vi "Sets the ACW voltage for MANU.vi"(5 "Enable to Query":bool, 7 "Enable to Setup":bool, 8 "error in":errorcluster, 10 "ACW voltage(kV)":sgl=0.1 min=0.1 max=5 format="%.3f", 11 "VISA resource name":refnum<visa-resource-name>) -> (0 "error out":errorcluster, 2 "Return ACW voltage":string, 3 "VISA resource name out":refnum<visa-resource-name>)   [LabVIEW 2011, in "GPT-9000.lvlib"]
uses:
  <instrlib>/GPT-9000/GPT-9000.lvlib
panel:
  # "kV"
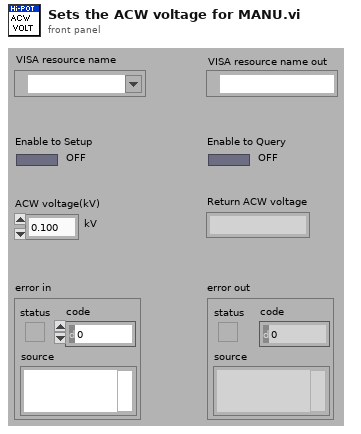
[diagram p1: front panel]
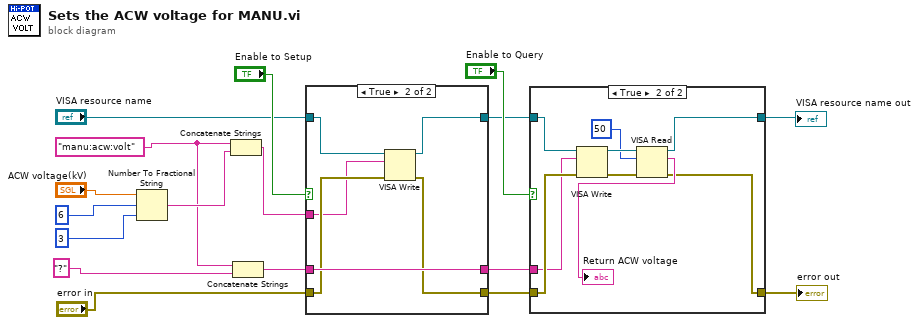
[diagram p0: block diagram]
diagram:
  w12 = "manu:acw:volt"
  n1 = Number To Fractional String(number="ACW voltage(kV)", width (-)=i16 6, precision (6)=i16 3) -> (F-format string=w16:string)  [unwired: 1 in]
  n2 = Concatenate Strings(w12, w16) -> (w10:string)
  n3 = Concatenate Strings(w12, "?") -> (w9:string)
  n4 = case shown="True" "Enable to Setup" {
    tunnel: w10 -> [_ w23]
    tunnel: w9 -> [w18 w26]
    tunnel: "error in" -> [w19 w24]
    tunnel: "VISA resource name" -> [w20 w25]
    tunnel: [w20 w22] -> w5
    tunnel: [w19 w21] -> w4
    tunnel: [w18 w26] -> w3
    frame False {
    }
    frame True {
      n5 = VISA Write(VISA resource name=w25, write buffer=w23, error in (no error)=w24) -> (VISA resource name out=w22:refnum<visa-resource-name>, error out=w21:errorcluster)  [unwired: 1 out]
    }
  }
  n6 = case shown="True" "Enable to Query" {
    tunnel: w5 -> [w28 w35]
    tunnel: w4 -> [w27 w34]
    tunnel: [w28 w30] -> w2
    tunnel: [w27 w29] -> w1
    tunnel: w3 -> [_ w33]
    frame False {
    }
    frame True {
      n7 = VISA Write(VISA resource name=w35, write buffer=w33, error in (no error)=w34) -> (VISA resource name out=w36:refnum<visa-resource-name>, error out=w37:errorcluster)  [unwired: 1 out]
      n8 = VISA Read(VISA resource name=w36, byte count=u32 50, error in (no error)=w37) -> (VISA resource name out=w30:refnum<visa-resource-name>, read buffer=→"Return ACW voltage":string, error out=w29:errorcluster)  [unwired: 1 out]
    }
  }
  "VISA resource name out" <- w2
  "error out" <- w1
